vi "New JSON ({String[]}).vi"(7 "keys":string[](array[string]), 8 "error in (no error)":errorcluster, 10 "values":string[](array[string])) -> (0 "error out":errorcluster, 3 "JSON Value out":refnum<class "JSON Value.lvclass">)   [LabVIEW 2016, in "JSON Value.lvclass"]
doc: "Create a new JSON Object initialized with the given key value pairs. The key and value arrays must be the same size."
uses:
  JSON Value.lvclass
  Object/Insert Value/Insert Value (Value[]).vi
  New JSON (String).vi
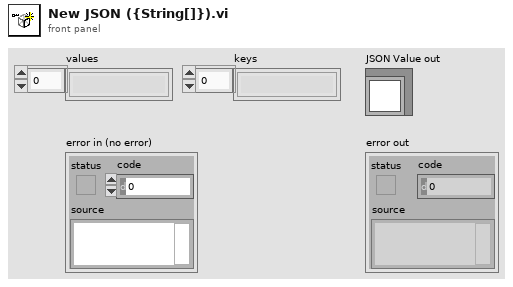
[diagram p1: front panel]
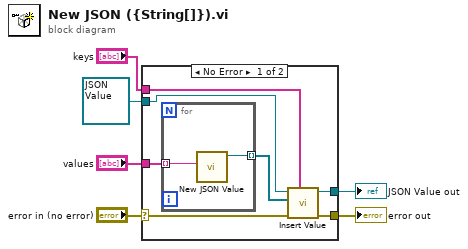
[diagram p0: block diagram]
diagram:
  n1 = case shown="No Error" "error in (no error)" {
    selector: "error in (no error)" -> [w13 w17]
    tunnel: [w12 w17] -> w5
    tunnel: [w10 w16] -> w4
    tunnel: refnum<class "JSON Value.lvclass"> refnum ("JSON out") -> [w11 w16]
    tunnel: "keys" -> [w9 _]
    tunnel: "values" -> [w8 _]
    frame No Error {
      n2 = for {
        tunnel: w8 -> [w15] mode=indexing
        tunnel: [w14] -> w7 mode=indexing
        n3 = call-poly "New JSON Value.vi"("value"=w15) -> ("JSON Value out"=w14:refnum<class "JSON Value.lvclass">)  [unwired: 9 in, 1 out]
      }
      n4 = call-poly "Insert Value.vi"("keys"=w9, "error in (no error)"=w13, "values"=w7, "JSON Value in"=w11) -> ("error out"=w12:errorcluster, "JSON Value out"=w10:refnum<class "JSON Value.lvclass">)  [unwired: 5 in, 1 out]
    }
    frame Error {
    }
  }
  "error out" <- w5
  "JSON Value out" <- w4
